vi "E Save as.vi"(0 "Excel._WorkBook":refnum<k7>, 5 "File path/保存路径":path, 7 "File path/保存名称":string, 11 "error in (no error)":errorcluster) -> (15 "error out":errorcluster)   [LabVIEW 2009]
doc: "将表格按指定的名称另存在指定的路径下并关闭此表格。"
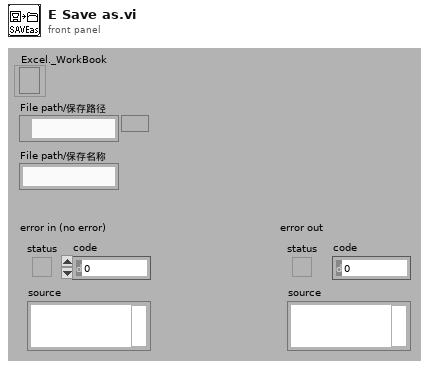
[diagram p1: front panel]
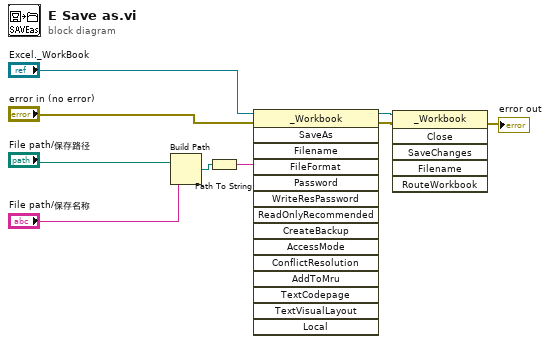
[diagram p0: block diagram]
diagram:
  n1 = Build Path(base path="File path/保存路径", name or relative path="File path/保存名称") -> (appended path=w7:path)
  n2 = Path To String(path=w7) -> (string=w6:string)
  n3 = invoke class="_Workbook" method="SaveAs"(reference="Excel._WorkBook", error in="error in (no error)", "Filename"=w6) -> (reference out=w4:refnum<k7>, error out=w2:errorcluster)  [unwired: 12 in, 13 out]
  n4 = invoke class="_Workbook" method="Close"(reference=w4, error in=w2) -> (error out=→"error out":errorcluster)  [unwired: 4 in, 5 out]
